vi "REM IO - Get Slave Data.vi"(8 "error in (no error)":errorcluster caption="Fehler (Eingang, kein Fehler)", 11 "EtherCAT Slave In":T9 {"VS ref" format="%.0x"}) -> (0 "error out":errorcluster caption="Fehler (Ausgang)", 3 "REM IO EtherCAT Slave":T1 {"I/O Output Data"."BD Refs"."Data Reference" format="%.0x"; "I/O Input Data"."BD Refs"."Data Reference" format="%.0x"; "I/O Output Vars"."VS ref" format="%.0x"; "I/O Imput Vars"."VS ref" format="%.0x"; "VS ref" format="%.0x"})   [LabVIEW 2016, in "Scan Engine Custom Device.lvlib"]
uses:
  Scan Engine Custom Device.lvlib
  <vilib>/NI Veristand/Custom Device API/Custom Device Item Ref.ctl
  Type Defs/REM IO ECAT Slave Data Cluster.ctl
  Type Defs/REM IO ECAT Slave IOV Cluster.ctl
  Type Defs/UDV Data Type.ctl
  Type Defs/Input Data.ctl
  <vilib>/NI Veristand/Custom Device API/Block Data Reference.ctl
  <vilib>/NI Veristand/Custom Device API/Data Reference.ctl
  Type Defs/Output Data.ctl
  Globals/Property Strings.vi
  <resource>/objmgr/IndComECAT.rc
  <vilib>/NI Veristand/Custom Device API/Custom Device API.lvlib
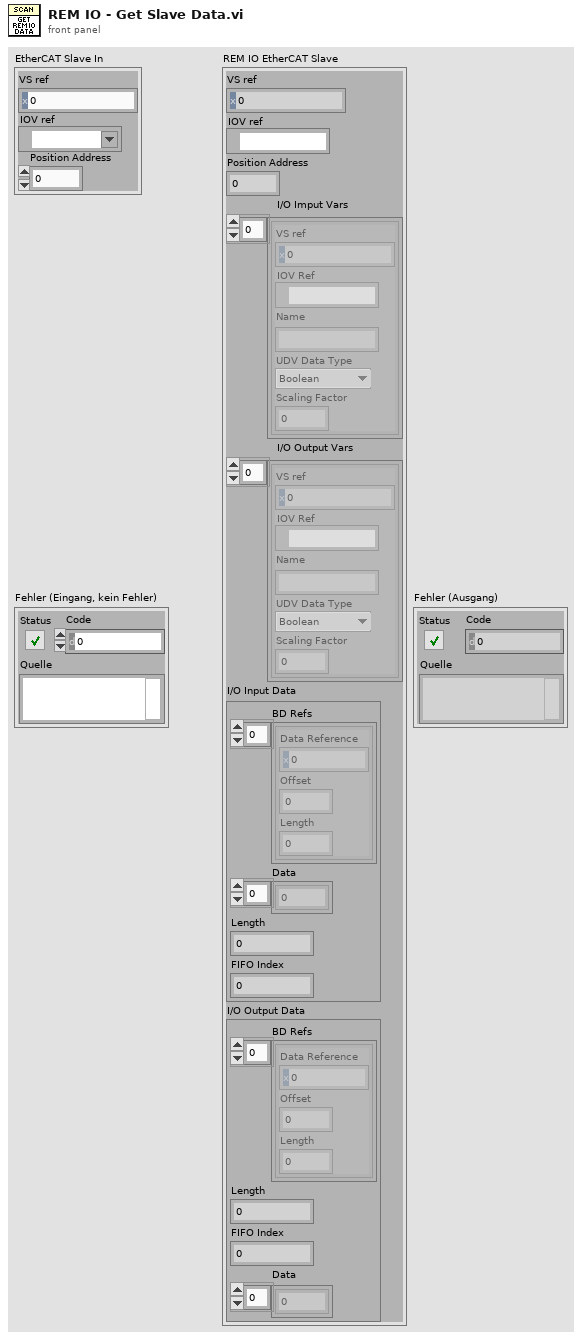
[diagram p1: front panel]
types:
  T1 = typedef "Scan Engine Custom Device.lvlib/REM IO ECAT Slave Data Cluster.ctl" = cluster{"VS ref":T2, "IOV ref":refnum<k21>, "Position Address":u16, "I/O Imput Vars ":T3[], "I/O Output Vars":T3[], "I/O Input Data":T5, "I/O Output Data":T8}
  T2 = typedef "Custom Device API.lvlib/Custom Device Item Ref.ctl" = u64
  T3 = typedef "Scan Engine Custom Device.lvlib/REM IO ECAT Slave IOV Cluster.ctl" = cluster{"VS ref":T2, "IOV Ref":refnum<k21>, "Name":string, "UDV Data Type":T4, "Scaling Factor":dbl}
  T4 = typedef "Scan Engine Custom Device.lvlib/UDV Data Type.ctl" = enum16{"Boolean", "Fixed Point", "Int8", "Int16", "Int32", "Int64", "U32 Bit Field", "UInt8", "UInt16", "UInt32", "UInt64", "Other"}
  T5 = typedef "Scan Engine Custom Device.lvlib/Input Data.ctl" = cluster{"BD Refs":T6[], "Data":dbl[], "Length":i32, "FIFO Index":i32}
  T6 = typedef "Custom Device API.lvlib/Block Data Reference.ctl" = cluster{"Data Reference":T7, "Offset":u64, "Length":u64}
  T7 = typedef "Custom Device API.lvlib/Data Reference.ctl" = i32
  T8 = typedef "Scan Engine Custom Device.lvlib/Output Data.ctl" = cluster{"BD Refs":T6[], "Length":i32, "FIFO Index":i32, "Data":dbl[]}
  T9 = cluster{"VS ref":T2, "IOV ref":refnum<k21>, "Position Address":u16}
  T10 = cluster{"Input VS Refs":T2[], "Output VS Refs":T2[]}
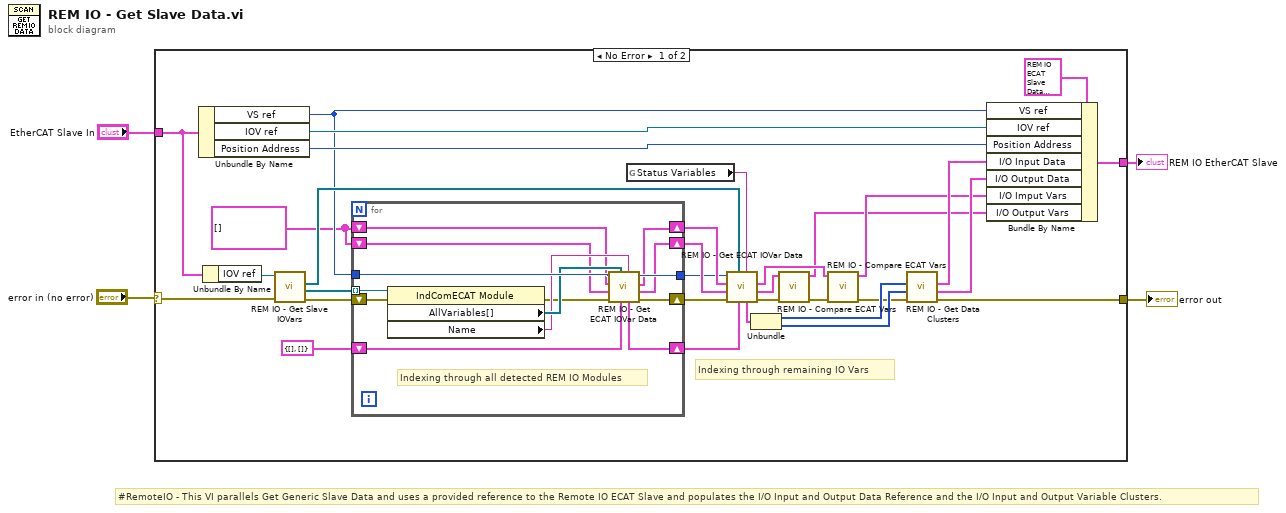
[diagram p0: block diagram]
diagram:
  # "#RemoteIO - This VI parallels Get Generic Slave Data and uses a provided reference to the Remote IO ECAT Slave and populates the I/O Input and Output Data Reference and the I/O Input and Output Variable Clusters."
  n1 = case shown="No Error" "error in (no error)" {
    selector: "error in (no error)" -> [w33 w51]
    tunnel: "EtherCAT Slave In" -> [w36 _]
    tunnel: [w21 w51] -> w3
    tunnel: [w15 _] -> w1
    frame No Error {
      w6 = T3[] [] ("I/O Input Vars Out")
      # "Indexing through remaining IO Vars"
      n2 = Unbundle By Name(w36) -> ("VS ref"=w17:T2, "IOV ref"=w34:refnum<k21>, "Position Address"=w35:u16)
      n3 = Unbundle By Name(w36) -> ("IOV ref"=w32:refnum<k21>)
      n4 = call "REM IO - Get Slave IOVars.vi"("error in (no error)"=w33, "ECAT Slave in"=w32) -> ("error IO"=w18:errorcluster, "REM IO Modules"=w20:refnum<k21>[], "ECAT Variablenobjekt"=w19:refnum<k21>[])  [unwired: 6 in, 1 out]
      n5 = for {
        shift-right: [w42] -> w27
        shift-left: w18 -> [w50]
        tunnel: w20 -> [w49] mode=indexing
        tunnel: w17 -> [w48]
        tunnel: [w45] -> w26
        shift-right: [w44] -> w29
        shift-left: w6 -> [w39]
        shift-right: [w43] -> w28
        shift-left: w6 -> [w38]
        shift-right: [w40] -> w16
        shift-left: T10 {"Input VS Refs"=[], "Output VS Refs"=[]} ("VS Refs Out") -> [w37]
        # "Indexing through all detected REM IO Modules"
        n6 = property class="IndComECAT Module"(reference=w49, error in=w50) -> (error out=w41:errorcluster, "AllVariables[]"=w47:refnum<k21>[], "Name"=w46:string)  [unwired: 1 out]
        n7 = call "REM IO - Get ECAT IOVar Data.vi"("Section Name"=w46, "VS Refs In"=w37, "ECAT Variablenobjekt"=w47, "error in (no error)"=w41, "I/O Output Vars In"=w38, "I/O Input Vars In"=w39, "VS ref"=w48) -> ("error out (Ausgang)"=w42:errorcluster, "I/O Output Vars Out"=w43:T3[], "I/O Input Vars Out"=w44:T3[], "VS ref 2"=w45:T2, "VS Refs Out"=w40:T10)
      }
      n8 = global read "Property Strings.vi" "Status Variables"() -> (w22:string)
      n9 = call "REM IO - Get ECAT IOVar Data.vi"("Section Name"=w22, "VS Refs In"=w16, "ECAT Variablenobjekt"=w19, "error in (no error)"=w27, "I/O Output Vars In"=w28, "I/O Input Vars In"=w29, "VS ref"=w26) -> ("error out (Ausgang)"=w11:errorcluster, "I/O Output Vars Out"=w12:T3[], "I/O Input Vars Out"=w13:T3[], "VS Refs Out"=w25:T10)  [unwired: 1 out]
      n10 = Unbundle(w25) -> ("Input VS Refs"=w24:T2[], "Output VS Refs"=w23:T2[])
      n11 = call "REM IO - Compare ECAT Vars.vi"("Fehler (Eingang, kein Fehler)"=w11, "I/O Vars In"=w12) -> ("Fehler (Ausgang)"=w14:errorcluster, "I/O Vars Out"=w7:T3[])  [unwired: 8 in]
      n12 = call "REM IO - Compare ECAT Vars.vi"("Fehler (Eingang, kein Fehler)"=w14, "I/O Vars In"=w13) -> ("Fehler (Ausgang)"=w10:errorcluster, "I/O Vars Out"=w8:T3[])  [unwired: 8 in]
      n13 = call "REM IO - Get Data Clusters.vi"("error in (no error)"=w10, "Output VS Refs"=w23, "Input VS Refs"=w24) -> ("error out"=w21:errorcluster, "I/O Output Data"=w30:T8, "I/O Input Data"=w31:T5)  [unwired: 6 in]
      n14 = Bundle By Name(cluster=T1 {"VS ref"=0, "IOV ref"="", "Position Address"=0, "I/O Imput Vars "=[], "I/O Output Vars"=[], "I/O Input Data"={"BD Refs"=[], "Data"=[], "Length"=0, "FIFO Index"=0}, "I/O Output Data"={"BD Refs"=[], "Length"=0, "FIFO Index"=0, "Data"=[]}} ("REM IO EtherCAT Slave"), "VS ref"=w17, "IOV ref"=w34, "Position Address"=w35, "I/O Input Data"=w31, "I/O Output Data"=w30, "I/O Imput Vars"=w8, "I/O Output Vars"=w7) -> (w15:T1)
    }
    frame Error {
    }
  }
  "error out" <- w3
  "REM IO EtherCAT Slave" <- w1
